vi "Index_string (SubVI).vi"(1 "Index(0..X)":i32, 4 "Physical Channel":tag="Dev1/ai0") -> (0 "Result":string)   [LabVIEW 2014]
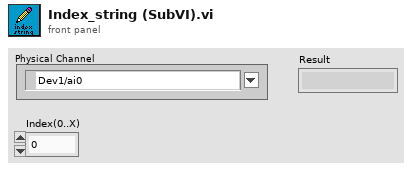
[diagram p1: front panel]
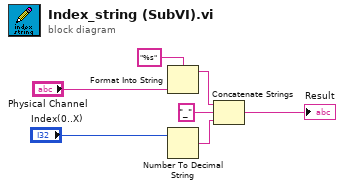
[diagram p0: block diagram]
diagram:
  n1 = Format Into String(format string="%s", "Physical Channel") -> (resulting string=w5:string)  [unwired: 2 in, 1 out]
  n2 = Number To Decimal String(number="Index(0..X)") -> (decimal integer string=w3:string)  [unwired: 1 in]
  n3 = Concatenate Strings(w5, "_" ("string"), w3) -> (→"Result":string)
